vi "Read Global.vi"(8 "error in (no error)":errorcluster, 9 "Semaphore Timeout":i32=-1) -> (0 "error out":errorcluster, 1 "Semaphore Timed Out":bool, 2 "DriveMotorsLeft Global":refnum<class "DriveMotorsLeft.lvclass">)   [LabVIEW 2013]
uses:
  DriveMotorsLeft.lvclass
  Robot Global Data.vi
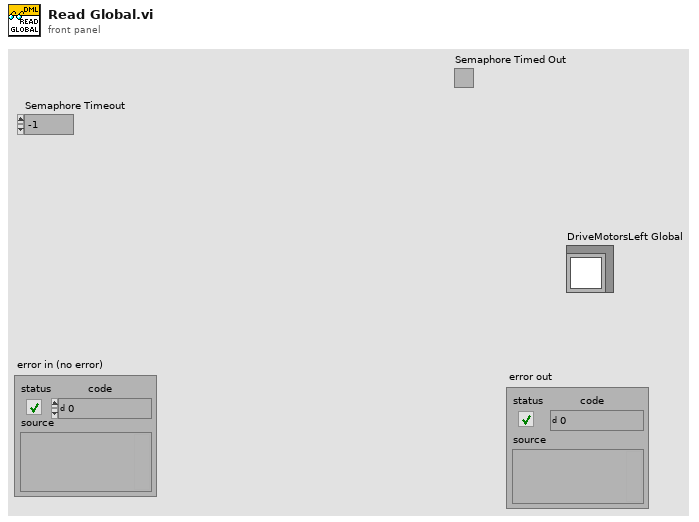
[diagram p1: front panel]
types:
  T1 = typedef "Semaphore RefNum" = refnum<k1>
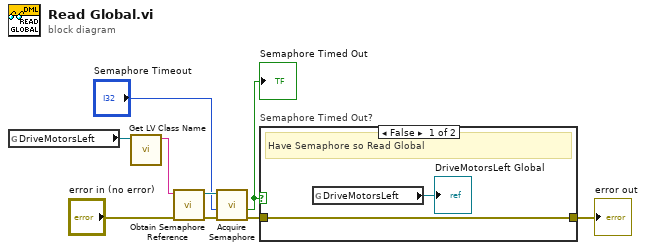
[diagram p0: block diagram]
diagram:
  n1 = global read "Robot Global Data.vi" "DriveMotorsLeft"() -> (w9:refnum<class "DriveMotorsLeft.lvclass">)
  n2 = call <vilib>:"Get LV Class Name.vi"("object"=w9) -> ("class name"=w8:string)  [unwired: 9 in, 1 out]
  n3 = call <vilib>:"Obtain Semaphore Reference.vi"("error in (no error)"="error in (no error)", "name (unnamed)"=w8) -> ("error out"=w6:errorcluster, "semaphore"=w7:T1)  [unwired: 3 in, 1 out]
  n4 = call <vilib>:"Acquire Semaphore.vi"("error in (no error)"=w6, "ms timeout (-1)"="Semaphore Timeout", "semaphore"=w7) -> ("error out"=w2:errorcluster, "timed out"=w4:bool)  [unwired: 2 in, 1 out]
  "Semaphore Timed Out" <- w4
  n5 = case "Semaphore Timed Out?" shown="False" w4 {
    tunnel: w2 -> [w10 w12]
    tunnel: [w10 w12] -> w1
    frame False {
      # "Have Semaphore so Read Global"
      n6 = global read "Robot Global Data.vi" "DriveMotorsLeft"() -> (→"DriveMotorsLeft Global":refnum<class "DriveMotorsLeft.lvclass">)
    }
    frame True {
      # "Don't read Global"
    }
  }
  "error out" <- w1
